vi "ESP_Full_State_Updated.vi"() -> ()   [LabVIEW 2021]
panel:
  out "Numeric":i32
  out "output array":sgl[][](array[numeric])
  out "Waveform Chart 2":sgl[][](graph)
  in  "stop streaming":bool
  in  "Shut dowm":bool
  in  "Full state":bool
  in  "Stream":bool
  in  "Re-zero":bool
  out "Waveform Chart":sgl[](graph)
  out "Stream on?":string
  out "Full state on?":string
  out "Full state":string
  # "Sampling rate is 225 Hz, please use the Setup software to change the rate"
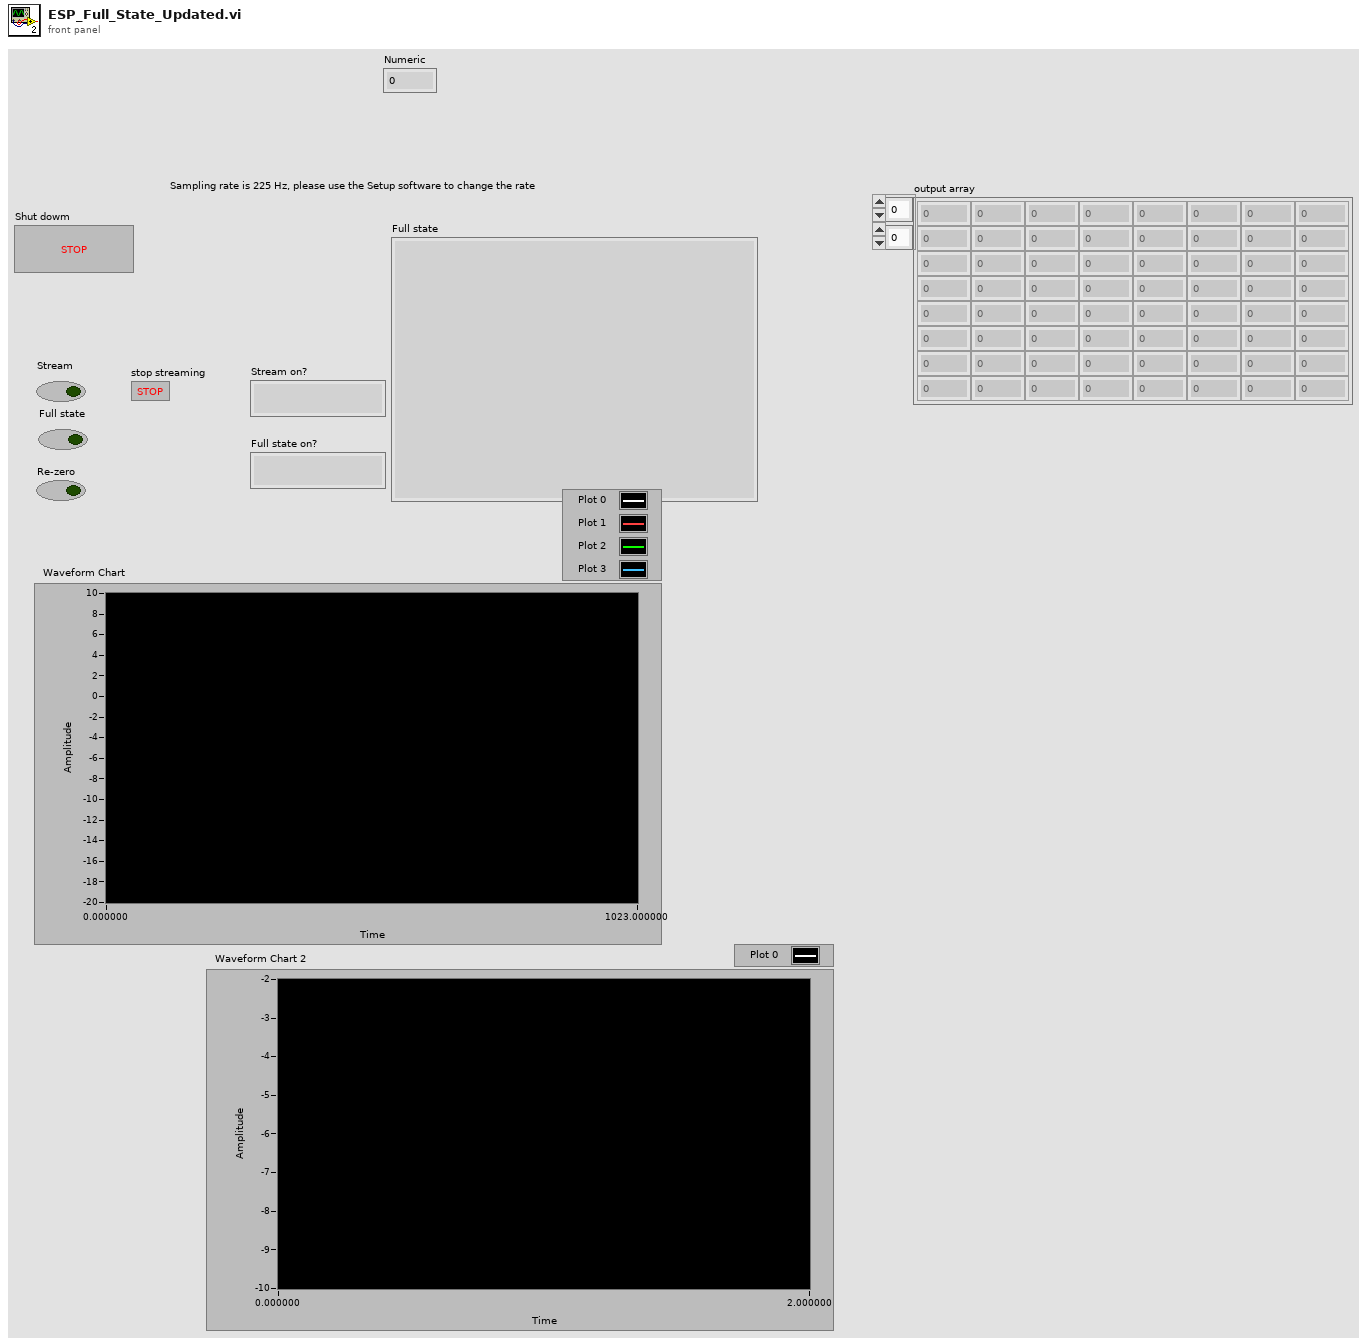
[diagram p1: front panel]
types:
  T1 = enum16{"Standard", "Buffered", "CRLF", "Immediate"}
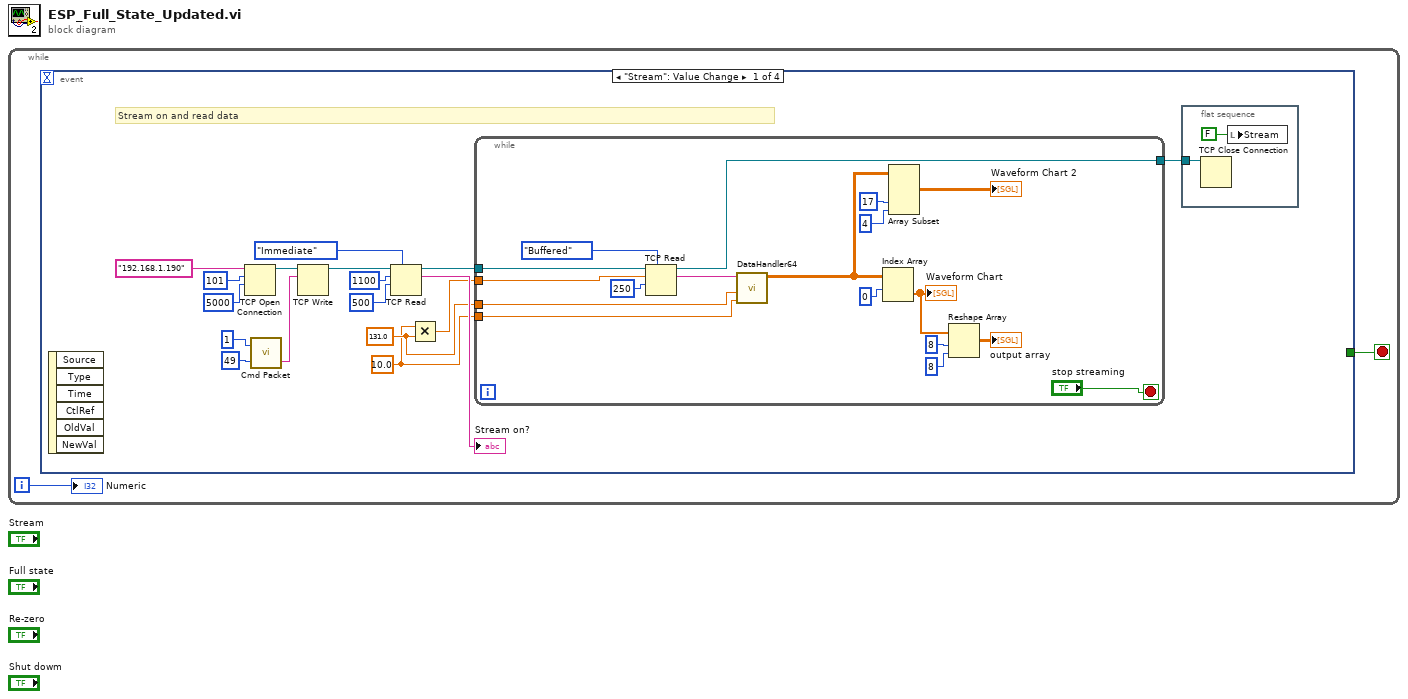
[diagram p0: block diagram]
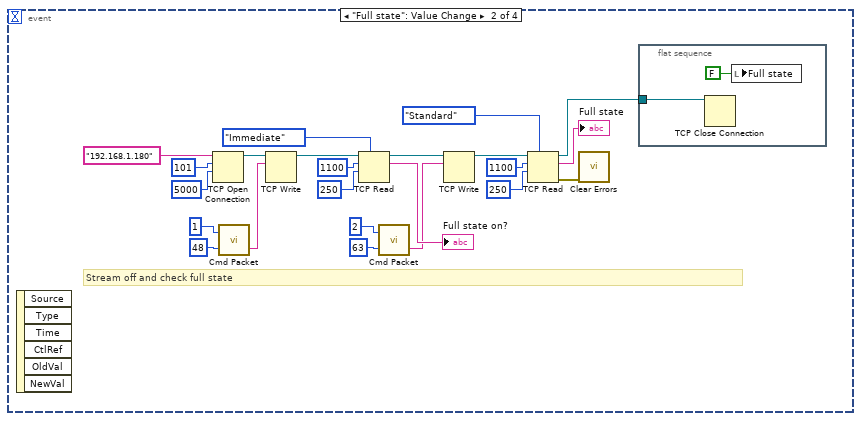
[diagram p2: hidden frame]
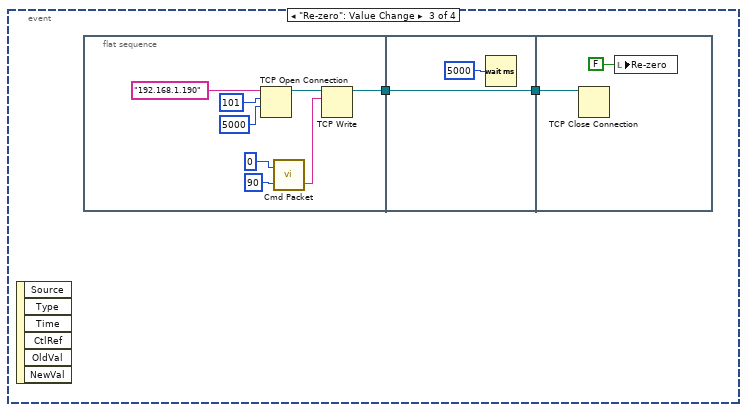
[diagram p3: hidden frame]
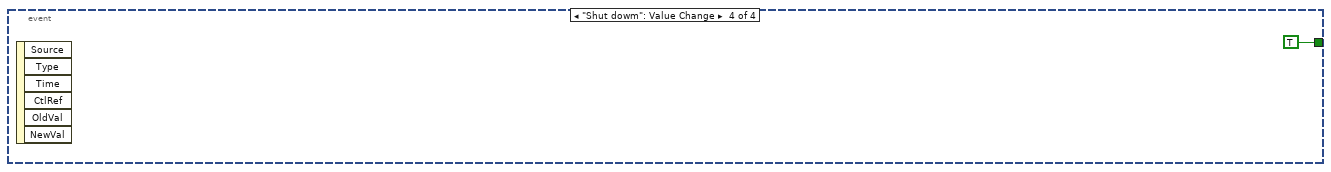
[diagram p4: hidden frame]
diagram:
  n1 = while {
    i -> [w1]
    stop <- w2 stop-if-true
    n2 = event shown="[0] \"Stream\": Value Change" {
      selector: _ -> [_ _ _ _]
      dyn-events: _ -> [_ _ _ _]
      timeout: _ -> [_ _ _ _]
      tunnel: [_ _ _ TRUE] -> w2
      event "Stream": Value Change {
        w3 = 10.0 ("Sampling Rate")
        w4 = 131.0 ("y")
        # "Stream on and read data"
        n3 = event-data() -> ()  [unwired: 1 in, 6 out]
        n4 = TCP Open Connection(address="192.168.1.190" ("Address"), remote port or service name=u16 101 ("Port"), timeout ms (60000)=5000) -> (connection ID=w13:refnum<k5>)  [unwired: 2 in, 1 out]
        n5 = call "Cmd Packet.vi"("Command Byte"=49 ("data in"), "Parameter Byte"=1 ("data in")) -> ("Command Packet Byte String"=w17:string)  [unwired: 1 out]
        n6 = TCP Write(connection ID=w13, data in=w17) -> (connection ID out=w15:refnum<k5>)  [unwired: 2 in, 2 out]
        n7 = TCP Read(connection ID=w15, bytes to read=1100, 7:T1."Immediate" ("mode (standard)"), 9:500 ("timeout ms (25000)")) -> (connection ID out=w18:refnum<k5>, data out=→"Stream on?":string)  [unwired: 1 in, 1 out]
        n8 = Multiply(x=w3, y=w4) -> (x*y=w14:dbl)
        n9 = while {
          tunnel: [w36] -> w19
          tunnel: w18 -> [w32]
          tunnel: w14 -> [w35]
          tunnel: w4 -> [w34]
          tunnel: w3 -> [w33]
          stop <- "stop streaming" stop-if-true
          n10 = TCP Read(connection ID=w32, bytes to read=w35, 7:T1."Buffered" ("mode (standard)"), 9:250 ("timeout ms (25000)")) -> (connection ID out=w36:refnum<k5>, data out=w39:string)  [unwired: 1 in, 1 out]
          n11 = call "DataHandler64.vi"("Data Cycles Per Buffer"=w33, "Rx Packet Byte size"=w34, "data out"=w39) -> ("Data"=w30:sgl[][])  [unwired: 2 in, 4 out]
          n12 = Index Array(array=w30, index (row)=0 ("Channel")) -> (element=w23:sgl[])  [unwired: 1 in]
          "Waveform Chart" <- w23
          n13 = Array Subset(array=w30, index (col)=17 ("index"), length (col)=4 ("length")) -> (→"Waveform Chart 2":sgl[][])  [unwired: 2 in]
          n14 = Reshape Array(w23, 8 ("dimension size"), 8 ("dimension size")) -> (→"output array":sgl[][])
        }
        n15 = flat-sequence {
          tunnel: w19 -> [w20]
          frame #0 {
            n16 = TCP Close Connection(connection ID=w20) -> ()  [unwired: 2 in, 2 out]
            n17 = local write "Stream"(FALSE) -> ()
          }
        }
      }
      event "Full state": Value Change {
        # "Stream off and check full state"
        n18 = event-data() -> ()  [unwired: 1 in, 6 out]
        n19 = TCP Open Connection(address="192.168.1.180" ("Address"), remote port or service name=u16 101 ("Port"), timeout ms (60000)=5000) -> (connection ID=w41:refnum<k5>)  [unwired: 2 in, 1 out]
        n20 = call "Cmd Packet.vi"("Command Byte"=48 ("data in"), "Parameter Byte"=u32 1 ("element")) -> ("Command Packet Byte String"=w58:string)  [unwired: 1 out]
        n21 = TCP Write(connection ID=w41, data in=w58) -> (connection ID out=w61:refnum<k5>)  [unwired: 2 in, 2 out]
        n22 = TCP Read(connection ID=w61, bytes to read=1100, 7:T1."Immediate" ("mode (standard)"), 9:250 ("timeout ms (25000)")) -> (connection ID out=w62:refnum<k5>, data out=→"Full state on?":string)  [unwired: 1 in, 1 out]
        n23 = call "Cmd Packet.vi"("Command Byte"=63 ("data in"), "Parameter Byte"=2 ("data in")) -> ("Command Packet Byte String"=w55:string)  [unwired: 1 out]
        n24 = TCP Write(connection ID=w62, data in=w55) -> (connection ID out=w56:refnum<k5>)  [unwired: 2 in, 2 out]
        n25 = TCP Read(connection ID=w56, bytes to read=1100, 7:T1."Standard" ("mode (standard)"), 9:250 ("timeout ms (25000)")) -> (connection ID out=w40:refnum<k5>, data out=→"Full state":string, error out=w59:errorcluster)  [unwired: 1 in]
        n26 = call <vilib>:"Clear Errors.vi"("error in (no error)"=w59) -> ()  [unwired: 5 in, 2 out]
        n27 = flat-sequence {
          tunnel: w40 -> [w64]
          frame #0 {
            n28 = TCP Close Connection(connection ID=w64) -> ()  [unwired: 2 in, 2 out]
            n29 = local write "Full state"(FALSE ("Full state")) -> ()
          }
        }
      }
      event "Re-zero": Value Change {
        n30 = event-data() -> ()  [unwired: 1 in, 6 out]
        n31 = flat-sequence {
          tunnel: [w67] -> w65
          tunnel: [w76] -> w66
          tunnel: w65 -> [w76]
          tunnel: w66 -> [w77]
          frame #0 {
            n32 = TCP Open Connection(address="192.168.1.190" ("Address"), remote port or service name=u16 101 ("Port"), timeout ms (60000)=5000) -> (connection ID=w74:refnum<k5>)  [unwired: 2 in, 1 out]
            n33 = call "Cmd Packet.vi"("Command Byte"=90 ("data in"), "Parameter Byte"=0 ("data in")) -> ("Command Packet Byte String"=w68:string)  [unwired: 1 out]
            n34 = TCP Write(connection ID=w74, data in=w68) -> (connection ID out=w67:refnum<k5>)  [unwired: 2 in, 2 out]
          }
          frame #1 {
            n35 = Wait (ms)(milliseconds to wait=u32 5000) -> ()  [unwired: 1 out]
          }
          frame #2 {
            n36 = TCP Close Connection(connection ID=w77) -> ()  [unwired: 2 in, 2 out]
            n37 = local write "Re-zero"(FALSE ("Re-zero")) -> ()
          }
        }
      }
      event "Shut dowm": Value Change {
        n38 = event-data() -> ()  [unwired: 1 in, 6 out]
      }
    }
    "Numeric" <- w1
  }
